vi "worksheet freeze panes opt.vi"(5 "type":u8, 6 "left_col":u16, 7 "top_row":u32, 8 "error in (no error)":errorcluster, 9 "first_col":u16, 10 "first_row":u32, 11 "worksheet":u32) -> (0 "error out":errorcluster)   [LabVIEW 8.6]
doc: "void worksheet_freeze_panes_opt(lxw_worksheet worksheet, lxw_row_t first_row, lxw_col_t first_col, lxw_row_t top_row, lxw_col_t left_col, uint8_t type);"
uses:
  pending_lvxlsxwriter/xlsxwriter.dll
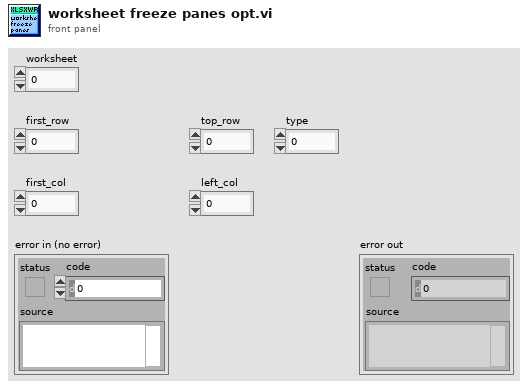
[diagram p1: front panel]
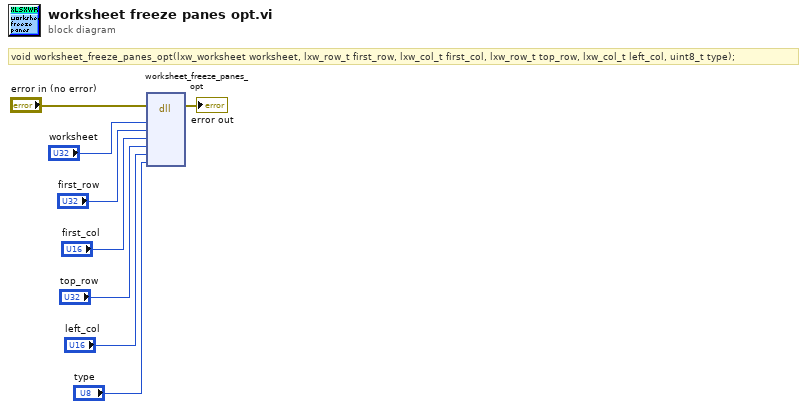
[diagram p0: block diagram]
diagram:
  # "void worksheet_freeze_panes_opt(lxw_worksheet worksheet, lxw_row_t first_row, lxw_col_t first_col, lxw_row_t top_row, lxw_col_t left_col, uint8_t type);"
  n1 = dll-call lib="C:/Users/WDAGUtilityAccount/Desktop/pending_lvxlsxwriter/xlsxwriter.*" fn="worksheet_freeze_panes_opt"(error in="error in (no error)", "worksheet"="worksheet", "first_row"="first_row", "first_col"="first_col", "top_row"="top_row", "left_col"="left_col", "type"="type") -> (error out=→"error out":errorcluster)  [unwired: 9 in, 1 out]
